vi "Data retrieve engine_SE.vi"(8 "error in (no error)":errorcluster, 10 "File Type":T3, 11 "Retrieve and Visualize":refnum<class "Retrieve and Visualize.lvclass">) -> (0 "error out":errorcluster, 3 "Retrieve and Visualize out":refnum<class "Retrieve and Visualize.lvclass">)   [LabVIEW 2020, in "Retrieve and Visualize.lvclass"]
uses:
  Retrieve and Visualize.lvclass
  <userlib>/LevyLab/LV-Data/LV-Data/Typedefs/File Type--enum.ctl
  Retrieve and Visualize.lvclass/Retrieve and Visualize.ctl
  <userlib>/LevyLab/XY Utilities/subVIs/Decimate (multiple).vi
  <userlib>/LevyLab/XY Utilities/subVIs/Decimate (single).vi
  <vilib>/Analysis/2dsp.llb/Decimate (single shot).vi
  <vilib>/Analysis/2dsp.llb/Decimate (single shot, DBL).vi
  <vilib>/Utility/error.llb/Error Cluster From Error Code.vi
  <vilib>/addons/WireFlow/_WF_ProgressBar.llb/ProgressBar_WireFlow.lvclass
  <userlib>/LevyLab/XY Utilities/xy_utilities.lvlib
  <userlib>/LevyLab/LV-Data/LV-Data/LV-Data.lvclass
panel:
  in  "Tab Control":T1(tab)=enum."Extracted data"
  out "Scan names":string[](array[string])
  out "Decimate point":dbl=1e-10 format="%#_1f"
  out "File or Folder Path":path=path "C:/Users/voodoo/Desktop/IV_separat_Vsgsweep_2fields_Vbg-2.8V"
  out "IV setup":T2={"# of Vslow"=1, "# Vfast"=1, "#IV Curves at each gate"=2, "B/T offset"=0, "Discard first # curves"=1, "Manual offset"=0}
  out "Portion of data":cluster{dbl, dbl}(slide)={0.75, 0.25} scale=0.0..1.0
  out "Extract paramaters from comments?":bool
  out "Gates and B":T4
  out "index":T5
  out "I vs V2T":cluster{dbl[], dbl[]}[](graph)
  out "V4T vs V2T":cluster{dbl[], dbl[]}[](graph)
  out "V4T vs V2T":cluster{dbl[], dbl[]}[][](array[cluster])
  out "Vslow":dbl[](array[numeric])
  out "Vfast":dbl[][](array[numeric])
  out "I vs V2T":cluster{dbl[], dbl[]}[][](array[cluster])
  out "Comments":string
  out "Vslowest":dbl
  # "Use to extract gate values in comments\neg. Vsg1="
  # "How many curves at each field/temperature? Usually should be N(Vslow)*N(Vfast)*N(each gate)"
  # "Discard first few IV curves at each gate if the gate need\ntime to settle"
  # "Default:\n4 terminal V vs I \n2 terminal V vs I"
  # "Default decimate on current axis instead of voltage axis. Decimation is needed for extracting dV/dI"
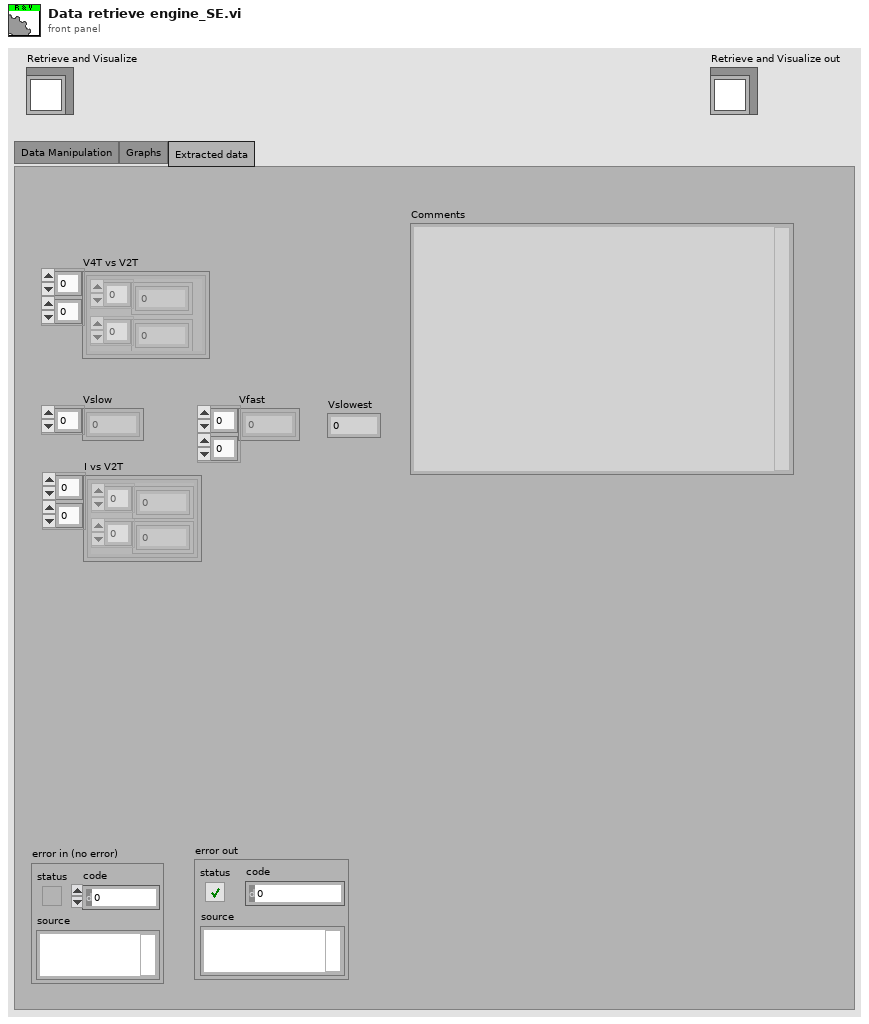
[diagram p1: front panel]
types:
  T1 = enum32{"Data Manipulation", "Graphs", "Extracted data"}
  T2 = cluster{"# of Vslow":i32, "# Vfast":i32, "#IV Curves at each gate":i32, "B/T offset":i32, "Discard first # curves":i32, "Manual offset":i32}
  T3 = typedef "LV-Data.lvclass/File Type--enum.ctl" = enum16{"DAT", "ITX", "TDMS", "VI"}
  T4 = cluster{"+X (V)":dbl, "+Y (V)":dbl, "-X (V)":dbl, "-Y (V)":dbl, "B (T)":dbl}
  T5 = cluster{"I-(A)":string, "I+(A)":string, "V4T+":string, "V4T-":string, "UG":string, "DG":string, "LG":string, "B":string, "Temperature":string, "Vfast":string, "Vslow":string}
  T6 = cluster{"UG":dbl, "DG":dbl, "LG":dbl, "B":dbl, "Temperature":dbl}
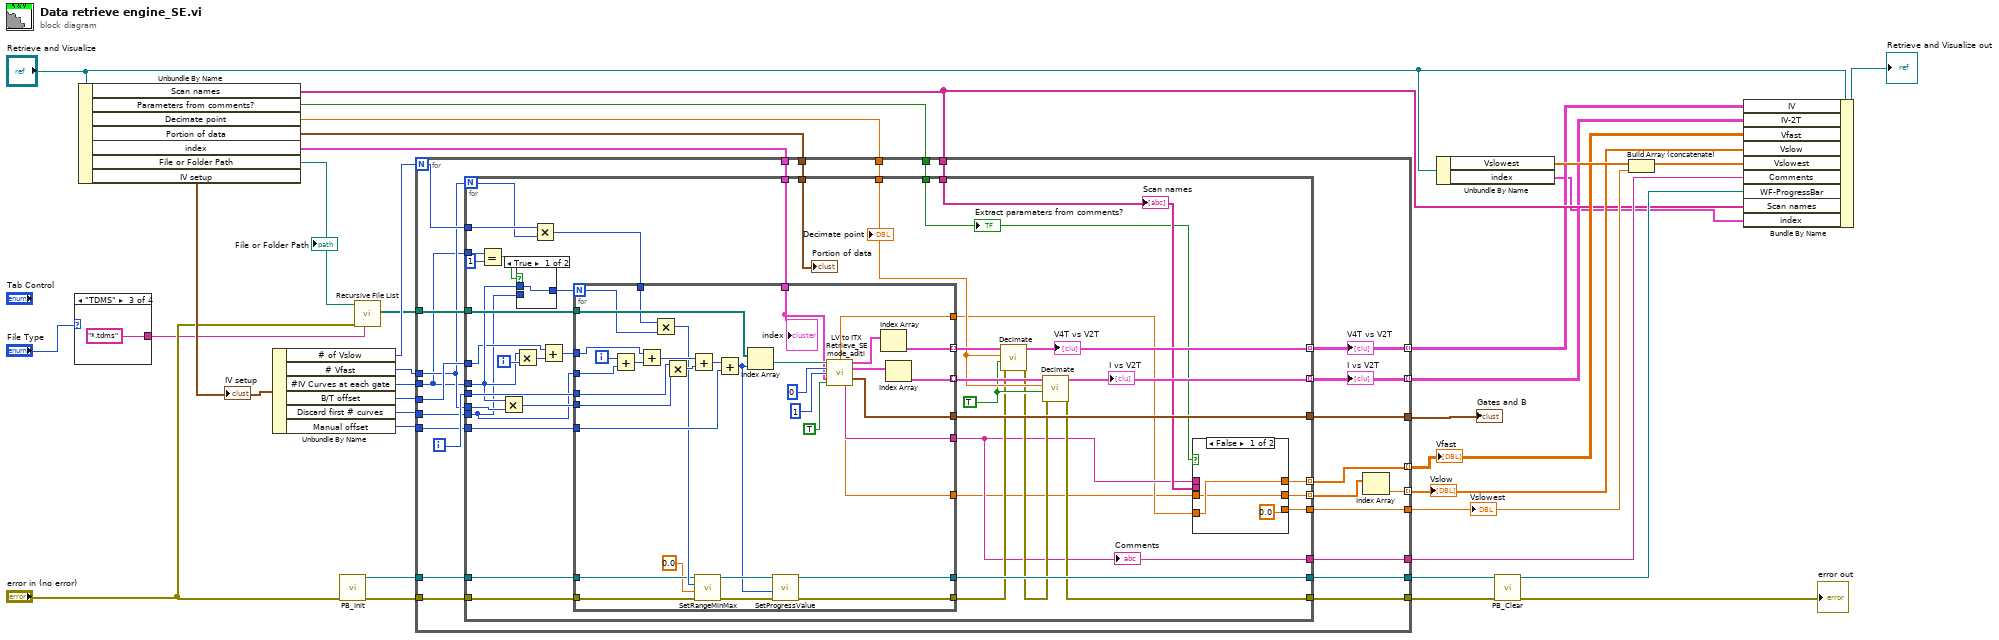
[diagram p0: block diagram]
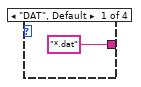
[diagram p2: hidden frame]
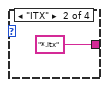
[diagram p3: hidden frame]
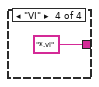
[diagram p4: hidden frame]
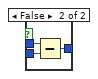
[diagram p5: hidden frame]
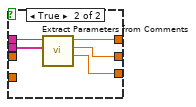
[diagram p6: hidden frame]
diagram:
  n1 = case shown="\"TDMS\"" "File Type" {
    tunnel: ["*.dat" ("pattern") "*.itx" ("pattern") "*.tdms" ("pattern") "*.vi" ("pattern")] -> w8
    frame "DAT", Default {
    }
    frame "ITX" {
    }
    frame "TDMS" {
    }
    frame "VI" {
    }
  }
  n2 = Unbundle By Name("Retrieve and Visualize") -> ("Scan names"=w7:string[], "Parameters from comments?"=w22:bool, "Decimate point"=w23:dbl, "Portion of data"=w24:cluster{dbl, dbl}, "index"=w25:T5, "File or Folder Path"=w27:path, "IV setup"=w26:T2)
  "File or Folder Path" <- w27
  "IV setup" <- w26
  n3 = Unbundle By Name(w26) -> ("# of Vslow"=w35:i32, "# Vfast"=w34:i32, "#IV Curves at each gate"=w33:i32, "B/T offset"=w31:i32, "Discard first # curves"=w32:i32, "Manual offset"=w30:i32)
  n4 = call <vilib>:"PB_Init.vi"("error in (no error)"="error in (no error)") -> ("error out"=w20:errorcluster, "WF-ProgressBar out"=w29:refnum<class "ProgressBar_WireFlow.lvclass">)  [unwired: 9 in]
  n5 = call <vilib>:"Recursive File List.vi"("pattern"=w8, "error in (no error)"="error in (no error)", "Folder Path"=w27) -> ("All Files in Dir"=w28:path[])  [unwired: 4 in, 4 out]
  n6 = for {
    N: w35 -> [w55]
    tunnel: [w63] -> w14 mode=indexing
    tunnel: w28 -> [w62]
    tunnel: w34 -> [w43]
    tunnel: w33 -> [w42]
    tunnel: w32 -> [w61]
    tunnel: w31 -> [w60]
    tunnel: w30 -> [w59]
    tunnel: [w41] -> w5 mode=indexing
    tunnel: [w40] -> w4 mode=indexing
    tunnel: [w57] -> w15 mode=indexing
    tunnel: [w56] -> w17
    tunnel: w29 -> [w54]
    tunnel: w25 -> [w53]
    tunnel: w24 -> [w52]
    tunnel: w23 -> [w51]
    tunnel: [w50] -> w6
    tunnel: [w49] -> w19
    tunnel: [w48] -> w13
    tunnel: w22 -> [w47]
    tunnel: w7 -> [w46]
    tunnel: w20 -> [w45]
    tunnel: [w44] -> w12
    i -> [w64]
    n7 = for {
      N: w43 -> [w91]
      tunnel: w43 -> [w101]
      tunnel: w64 -> [w100]
      tunnel: [w94] -> w50
      tunnel: w62 -> [w99]
      tunnel: w42 -> [w98]
      tunnel: w61 -> [w77]
      tunnel: w60 -> [w97]
      tunnel: w59 -> [w96]
      tunnel: [w93] -> w56
      tunnel: [w95] -> w58 mode=indexing
      tunnel: [w67] -> w57 mode=indexing
      tunnel: w55 -> [w92]
      tunnel: w54 -> [w89]
      tunnel: w53 -> [w88]
      tunnel: w52 -> [w85]
      tunnel: w51 -> [w81]
      tunnel: [w68] -> w49
      tunnel: [w87] -> w48
      tunnel: w47 -> [w69]
      tunnel: w46 -> [w70]
      tunnel: w45 -> [w86]
      tunnel: [w71] -> w44
      tunnel: [w79] -> w41 mode=indexing
      tunnel: [w78] -> w40 mode=indexing
      tunnel: w42 -> [w76]
      i -> [w104]
      w80 = TRUE ("averaging (off)")
      n8 = Equal?(x=w76, y=1) -> (x = y?=w74:bool)
      n9 = Multiply(x=w98, y=w101) -> (x*y=w102:i32)
      n10 = Multiply(x=w98, y=w104) -> (x*y=w105:i32)
      n11 = case shown="True" w74 {
        tunnel: w98 -> [w106 w109]
        tunnel: [w106 w108] -> w84
        tunnel: w77 -> [_ w107]
        frame True {
        }
        frame False {
          n12 = Subtract(x=w109, y=w107) -> (x-y=w108:i32)
        }
      }
      n13 = Multiply(x=w92, y=w91) -> (x*y=w90:i32)
      n14 = Add(x=w97, y=w105) -> (x+y=w103:i32)
      n15 = for {
        N: w84 -> [w137]
        tunnel: w103 -> [w152]
        tunnel: [w128] -> w68
        tunnel: w102 -> [w122]
        tunnel: [w149] -> w83 mode=indexing
        tunnel: w100 -> [w147]
        tunnel: [w121] -> w94
        tunnel: w77 -> [w146]
        tunnel: [w145] -> w82 mode=indexing
        tunnel: w99 -> [w144]
        tunnel: w96 -> [w142]
        tunnel: w90 -> [w138]
        tunnel: w89 -> [w135]
        tunnel: w88 -> [w118]
        tunnel: [w127] -> w87
        tunnel: w86 -> [w126]
        tunnel: [w124] -> w73
        tunnel: [w120] -> w66
        tunnel: [w119] -> w65
        i -> [w139]
        n16 = Add(x=w139, y=w146) -> (x+y=w148:i32)
        n17 = Add(x=w152, y=w148) -> (x+y=w151:i32)
        n18 = Multiply(x=w138, y=w137) -> (x*y=w136:i32)
        n19 = Multiply(x=w147, y=w122) -> (x*y=w150:i32)
        n20 = Add(x=w151, y=w150) -> (x+y=w143:i32)
        n21 = call-dynamic "SetRangeMinMax.vi"("error in (no error)"=w126, "Min (0)"=0.0, "Max (1)"=w136, "WF-ProgressBar in"=w135) -> ("error out"=w125:errorcluster, "WF-ProgressBar out"=w133:refnum<class "ProgressBar_WireFlow.lvclass">)  [unwired: 6 in]
        n22 = Add(x=w143, y=w142) -> (x+y=w132:i32)
        n23 = Index Array(array=w144, index=w132) -> (element=w123:path)
        n24 = call-dynamic "SetProgressValue.vi"("error in (no error)"=w125, "Value"=w132, "WF-ProgressBar in"=w133) -> ("error out"=w124:errorcluster, "WF-ProgressBar out"=w127:refnum<class "ProgressBar_WireFlow.lvclass">)  [unwired: 6 in, 1 out]
        n25 = call "LV to ITX Retrieve_SE mode_aditi.vi"("File or Folder Path"=w123, "offset"=0, "length"=1, "index"=w118, "stop"=TRUE) -> ("Vfast"=w120:dbl, "Vslow"=w119:dbl, "V4T vs V2T"=w141:cluster{dbl[], dbl[]}[], "I vs V2T"=w140:cluster{dbl[], dbl[]}[], "Gates, B and T"=w121:T6, "Comments"=w128:string)  [unwired: 4 in, 1 out]
        n26 = Index Array(array=w141) -> (element=w149:cluster{dbl[], dbl[]})  [unwired: 1 in]
        n27 = Index Array(array=w140) -> (element=w145:cluster{dbl[], dbl[]})  [unwired: 1 in]
        "index" <- w118
      }
      "Comments" <- w68
      n28 = call-poly <userlib>:"Decimate.vi"("error in (no error)"=w73, "averaging (off)"=w80, "decimating factor (1)"=w81, "XY-data"=w83) -> ("error out"=w72:errorcluster, "Decimated XY-data out"=w79:cluster{"X-array":dbl[], "Y-array":dbl[]}[])  [unwired: 6 in]
      "V4T vs V2T" <- w79
      n29 = call-poly <userlib>:"Decimate.vi"("error in (no error)"=w72, "averaging (off)"=w80, "decimating factor (1)"=w81, "XY-data"=w82) -> ("error out"=w71:errorcluster, "Decimated XY-data out"=w78:cluster{"X-array":dbl[], "Y-array":dbl[]}[])  [unwired: 6 in]
      "I vs V2T" <- w78
      n30 = case shown="False" w69 {
        tunnel: [w111 w117] -> w67
        tunnel: [0.0 ("Numeric 3") w116] -> w93
        tunnel: [w110 w115] -> w95
        tunnel: w70 -> [_ w114]
        tunnel: w68 -> [_ w113]
        tunnel: w66 -> [w111 _]
        tunnel: w65 -> [w110 _]
        frame False {
        }
        frame True {
          n31 = call "Extract Parameters from Comments.vi"("Scan names"=w114, "Comments"=w113) -> ("Numeric 3"=w116:dbl, "Numeric 2"=w115:dbl, "Numeric 1"=w117:dbl)  [unwired: 7 in]
        }
      }
      "Portion of data" <- w85
      "Decimate point" <- w81
      "Scan names" <- w70
      "Extract paramaters from comments?" <- w69
    }
    "V4T vs V2T" <- w41
    "I vs V2T" <- w40
    n32 = Index Array(array=w58) -> (element=w63:dbl)  [unwired: 1 in]
  }
  "Vslow" <- w14
  "Vfast" <- w15
  "Vslowest" <- w17
  "Gates and B" <- w6
  n33 = Unbundle By Name("Retrieve and Visualize") -> ("Vslowest"=w16:dbl[], "index"=w1:T5)
  n34 = call-dynamic "PB_Clear.vi"("error in (no error)"=w12, "WF-ProgressBar in"=w13) -> ("error out"=→"error out":errorcluster, "WF-ProgressBar out"=w11:refnum<class "ProgressBar_WireFlow.lvclass">)  [unwired: 8 in]
  n35 = Build Array (concatenate)(w16, w17) -> (w18:dbl[])
  n36 = Bundle By Name(cluster="Retrieve and Visualize", "IV"=w5, "IV-2T"=w4, "Vfast"=w15, "Vslow"=w14, "Vslowest"=w18, "Comments"=w19, "WF-ProgressBar"=w11, "Scan names"=w7, "index"=w1) -> (→"Retrieve and Visualize out":refnum<class "Retrieve and Visualize.lvclass">)
